vi "Log.vi"(8 "error in (no error)":errorcluster, 10 "String":string, 11 "Logger in":refnum<class "Logger.lvclass">) -> (0 "error out":errorcluster, 3 "Logger out":refnum<class "Logger.lvclass">)   [LabVIEW 2020, in "Logger.lvlib" / "Logger.lvclass"]
uses:
  Logger.lvclass
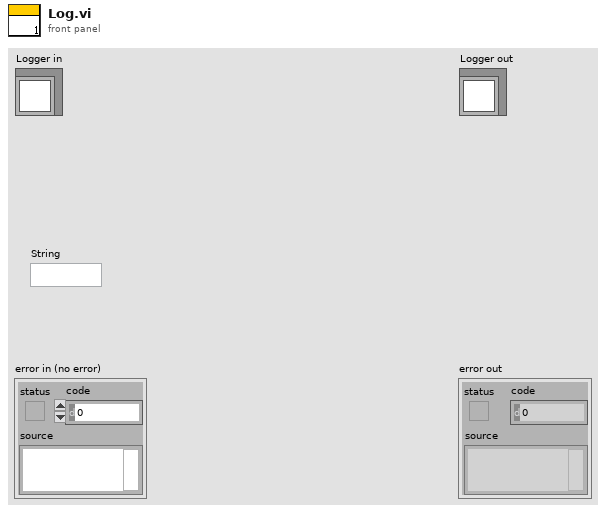
[diagram p1: front panel]
types:
  T1 = enum16{"open", "replace", "create", "open or create", "replace or create", "replace or create with confirmation"}
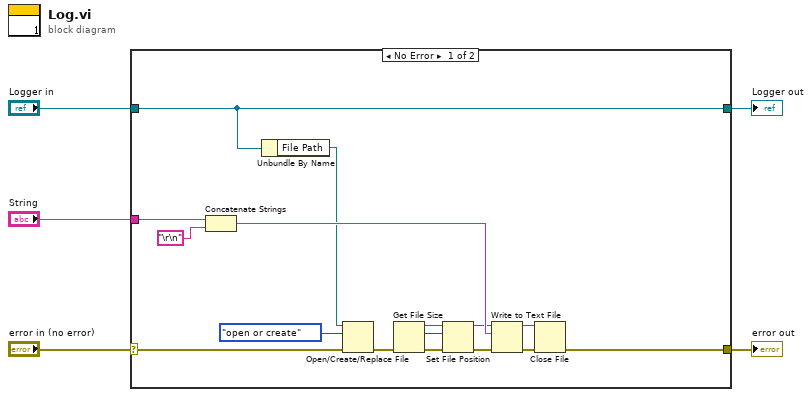
[diagram p0: block diagram]
diagram:
  n1 = case shown="No Error" "error in (no error)" {
    selector: "error in (no error)" -> [w14 w23]
    tunnel: [w13 w23] -> w4
    tunnel: [w8 w22] -> w2
    tunnel: "Logger in" -> [w8 w22]
    tunnel: "String" -> [w11 _]
    frame No Error {
      n2 = Concatenate Strings(w11, "\r\n") -> (w10:string)
      n3 = Unbundle By Name(w8) -> ("File Path"=w7:path)
      n4 = Open/Create/Replace File(file path (use dialog)=w7, error in=w14, operation (0:open)=T1."open or create") -> (error out=w21:errorcluster)  [unwired: 3 in, 2 out]
      n5 = Get File Size(error in=w21) -> (refnum out=w20:refnum<file>, size (in bytes)=w18:i64, 0:w19:errorcluster)  [unwired: 1 in]
      n6 = Set File Position(offset (in bytes) (0)=w18, refnum=w20, error in=w19) -> (refnum out=w9:refnum<file>, error out=w17:errorcluster)  [unwired: 1 in]
      n7 = Write to Text File(file (use dialog)=w9, text=w10, error in=w17) -> (refnum out=w15:refnum<file>, error out=w16:errorcluster)  [unwired: 1 in, 1 out]
      n8 = Close File(refnum=w15, error in=w16) -> (error out=w13:errorcluster)  [unwired: 1 out]
    }
    frame Error {
    }
  }
  "error out" <- w4
  "Logger out" <- w2
